vi "rqcBob Configure PD Detect FIFO (2PD).vi"(8 "error in":errorcluster, 9 "PD.detect fifo depth":u32=1000000, 10 "PD.detect fifo write enable":bool, 11 "FPGA reference in":refnum<k20>) -> (0 "error out":errorcluster, 3 "FPGA reference out":refnum<k20>)   [LabVIEW 2018]
uses:
  <vilib>/Utility/error.llb/Error Cluster From Error Code.vi
  <vilib>/rvi/errors/niLvFpgaAdjustHostInterfaceError.vi
  <vilib>/rvi/interface/common/niFpgaWaitOnOcc.vi
  <vilib>/rvi/interface/nirviReadWriteControl/nirviReadWriteControl.xnode
  <vilib>/rvi/interface/nirviMethod/nirviMethod.xnode
  <vilib>/rvi/errors/niLvFpgaMergeErrorWithErrorCode.vi
  <vilib>/FPGAPlugInAG/Dynamic/niLvFpga_StartFifo_Dynamic.vi
  <vilib>/FPGAPlugInAG/Dynamic/niLvFpga_ConfigureFifo_Dynamic.vi
  NiFpgaLv.dll
  <vilib>/rvi/interface/Simulation/niFpgaSimulationCallBeginRW.vi
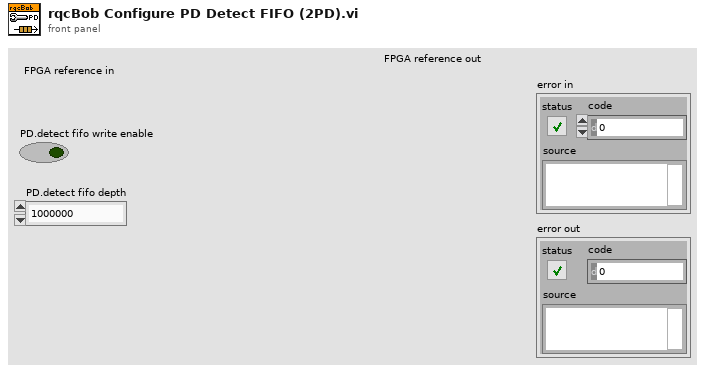
[diagram p1: front panel]
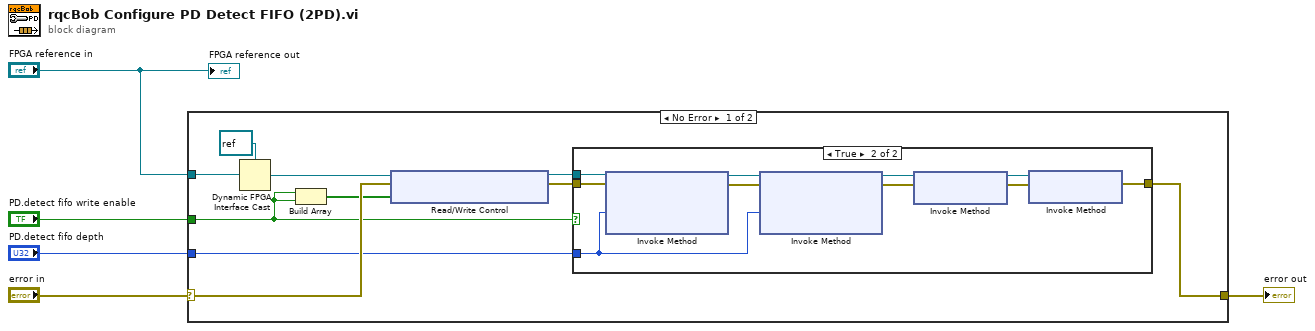
[diagram p0: block diagram]
diagram:
  n1 = case shown="No Error" "error in" {
    selector: "error in" -> [w15 w27]
    tunnel: [w9 w27] -> w3
    tunnel: "FPGA reference in" -> [w13 _]
    tunnel: "PD.detect fifo write enable" -> [w6 _]
    tunnel: "PD.detect fifo depth" -> [w8 _]
    frame No Error {
      n2 = Dynamic FPGA Interface Cast(Session In=refnum<k20> refnum ("FPGA Interface"), Type=w13) -> (Session Out=w12:refnum<k20>)
      n3 = Build Array(w6, w6) -> (w7:bool[])
      n4 = xnode "Read/Write Control"("FPGA VI Reference In"=w12, "error in"=w15, "PD.detect fifo write enable"=w7) -> ("FPGA VI Reference Out"=w11:refnum<k20>, "error out"=w10:errorcluster)
      n5 = case shown="True" w6 {
        tunnel: w11 -> [_ w26]
        tunnel: w10 -> [w16 w25]
        tunnel: [w16 w24] -> w9
        tunnel: w8 -> [_ w21]
        frame False {
        }
        frame True {
          n6 = xnode "Invoke Method"("FPGA VI Reference In"=w26, "error in"=w25, "Requested Depth"=w21) -> ("FPGA VI Reference Out"=w23:refnum<k20>, "error out"=w22:errorcluster)  [unwired: 1 out]
          n7 = xnode "Invoke Method"("FPGA VI Reference In"=w23, "error in"=w22, "Requested Depth"=w21) -> ("FPGA VI Reference Out"=w18:refnum<k20>, "error out"=w17:errorcluster)  [unwired: 1 out]
          n8 = xnode "Invoke Method"("FPGA VI Reference In"=w18, "error in"=w17) -> ("FPGA VI Reference Out"=w20:refnum<k20>, "error out"=w19:errorcluster)
          n9 = xnode "Invoke Method"("FPGA VI Reference In"=w20, "error in"=w19) -> ("error out"=w24:errorcluster)  [unwired: 1 out]
        }
      }
    }
    frame Error {
    }
  }
  "error out" <- w3
  "FPGA reference out" <- "FPGA reference in"
